vi "CheckBottomRight.vi"(0 "Chessboard":T2, 5 "ItemIndex":T1, 7 "StoneColor":u16, 11 "error in (no error)":errorcluster) -> (15 "error out":errorcluster)   [LabVIEW 2009]
uses:
  Controls/Chess.ctl
  Controls/ItemIndex.ctl
  BottomRightHaveSameStone.vi
  Controls/directions.ctl
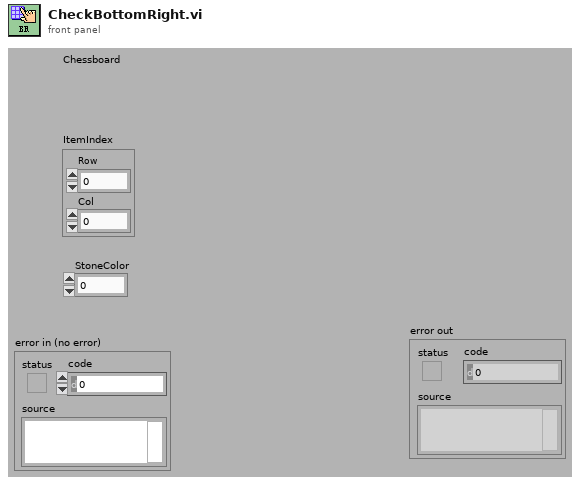
[diagram p1: front panel]
types:
  T1 = typedef "ItemIndex.ctl" = cluster{"Row":i32, "Col":i32}
  T2 = typedef "Chess.ctl" = u16[][]
  T3 = typedef "directions.ctl" = enum16{"Left", "Right", "Top", "Bottom", "TopLeft", "TopRight", "BottomLeft", "BottomRight", "ClearAll", "ReadAll"}
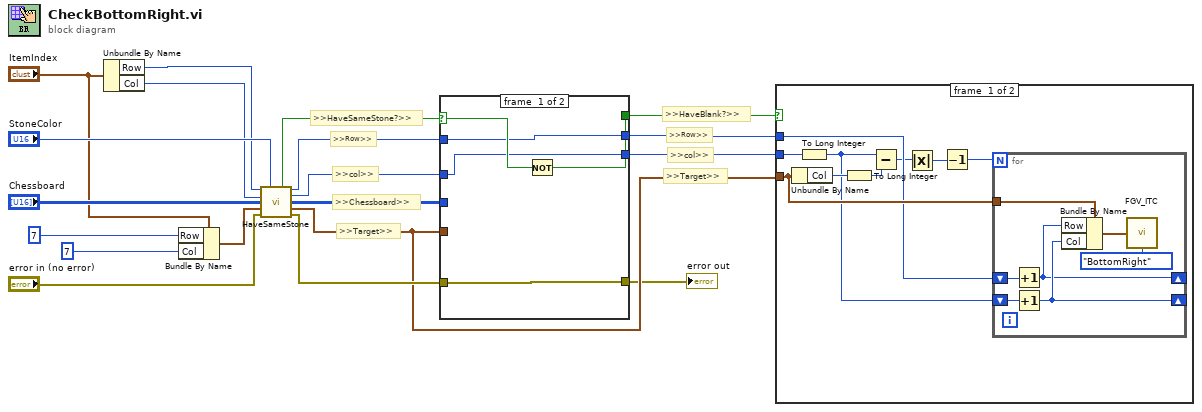
[diagram p0: block diagram]
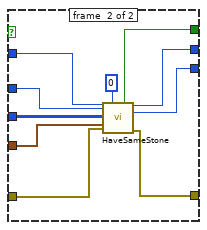
[diagram p3: hidden frame]
diagram:
  # ">>HaveBlank?>>"
  # ">>HaveSameStone?>>"
  # ">>Target>>"
  # ">>col>>"
  # ">>Row>>"
  # ">>Target>>"
  # ">>Chessboard>>"
  # ">>col>>"
  # ">>Row>>"
  n1 = Unbundle By Name("ItemIndex") -> ("Row"=w15:i32, "Col"=w3:i32)
  n2 = Bundle By Name(cluster="ItemIndex", "Row"=u32 7 ("Col"), "Col"=u32 7) -> (w14:T1)
  n3 = call-poly "HaveSameStone.vi"("Row in"=w15, "StoneColor"="StoneColor", "Col in"=w3, "Chessboard"="Chessboard", "TatgetIndex"=w14, "error in (no error)"="error in (no error)") -> ("HaveSameStone?"=w12:bool, "Row out"=w10:i32, "Col out"=w11:i32, "Chessboard out"=w13:T2, "SSIndex"=w6:T1, "error out"=w9:errorcluster)  [unwired: 4 in]
  n4 = case shown="True" w12 {
    selector: w12 -> [w24 _]
    tunnel: w6 -> [_ w33]
    tunnel: w13 -> [_ w32]
    tunnel: w11 -> [w20 w31]
    tunnel: w10 -> [w21 w30]
    tunnel: w9 -> [w22 w29]
    tunnel: [w23 w28] -> w8
    tunnel: [w22 w27] -> w5
    tunnel: [w21 w26] -> w7
    tunnel: [w20 w25] -> w1
    frame #0 {
      n5 = Not(x=w24) -> (.not. x?=w23:bool)
    }
    frame #1 {
      n6 = call-poly "HaveSameStone.vi"("Row in"=w30, "StoneColor"=u16 0, "Col in"=w31, "Chessboard"=w32, "TatgetIndex"=w33, "error in (no error)"=w29) -> ("HaveSameStone?"=w28:bool, "Row out"=w26:i32, "Col out"=w25:i32, "error out"=w27:errorcluster)  [unwired: 4 in, 2 out]
    }
  }
  "error out" <- w5
  n7 = case shown="False" w8 {
    tunnel: w7 -> [w42 _]
    tunnel: w1 -> [w39 _]
    tunnel: w6 -> [w43 _]
    frame #0 {
      n8 = Unbundle By Name(w43) -> ("Col"=w40:i32)
      n9 = To Long Integer(number=w39) -> (32bit integer=w38:i32)
      n10 = To Long Integer(number=w40) -> (32bit integer=w41:i32)
      n11 = Subtract(x=w38, y=w41) -> (x-y=w37:i32)
      n12 = Absolute Value(x=w37) -> (abs(x)=w36:i32)
      n13 = Decrement(x=w36) -> (x-1=w35:i32)
      n14 = for {
        N: w35 -> [_]
        shift-right: [w48] -> _
        shift-left: w38 -> [w50]
        tunnel: w43 -> [w49]
        shift-right: [w44] -> _
        shift-left: w42 -> [w45]
        n15 = Increment(x=w45) -> (x+1=w44:i32)
        n16 = Increment(x=w50) -> (x+1=w48:i32)
        n17 = Bundle By Name(cluster=w49, "Row"=w44, "Col"=w48) -> (w47:T1)
        n18 = call "FGV_ITC.vi"("ItemIndex"=w47, "Action"=directions."BottomRight") -> ()  [unwired: 12 in, 2 out]
      }
    }
    frame #1 {
    }
  }
